vi "Threshold_Check.vi"(8 "error in (no error)":errorcluster, 11 "Simulators":T1 {"Milk Level" scale=0.0..100.0; "Bean Level" scale=0.0..100.0; "Water Level" scale=0.0..100.0}) -> (0 "error out":errorcluster, 2 "Success?":bool, 3 "Status":string)   [LabVIEW 2026]
uses:
  controls/Simulators.ctl
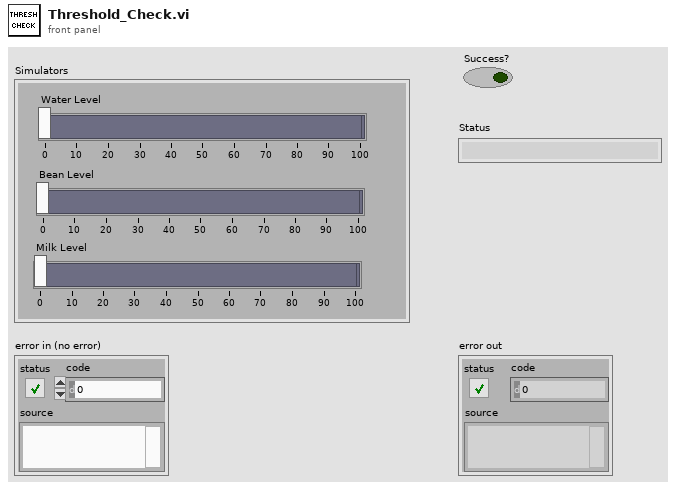
[diagram p1: front panel]
types:
  T1 = typedef "Simulators.ctl" = cluster{"Water Level":dbl, "Bean Level":dbl, "Milk Level":dbl}
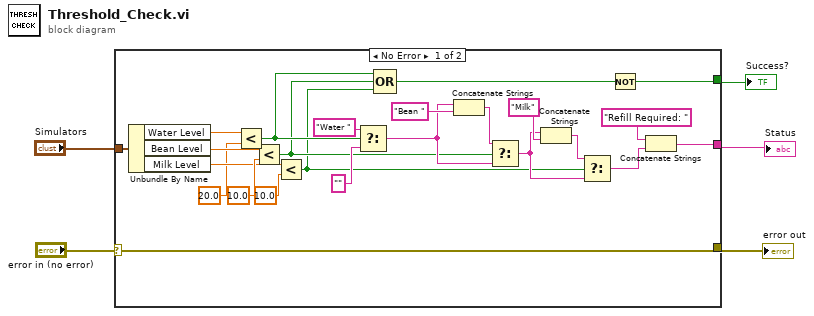
[diagram p0: block diagram]
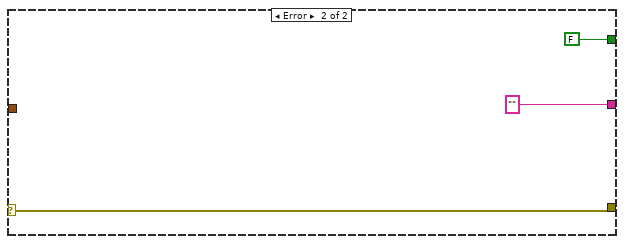
[diagram p2: hidden frame]
diagram:
  n1 = case shown="No Error" "error in (no error)" {
    selector: "error in (no error)" -> [w22 w32]
    tunnel: "Simulators" -> [w25 _]
    tunnel: [w22 w32] -> w3
    tunnel: [w11 ""] -> w2
    tunnel: [w6 FALSE] -> w1
    frame No Error {
      n2 = Unbundle By Name(w25) -> ("Water Level"=w24:dbl, "Bean Level"=w26:dbl, "Milk Level"=w27:dbl)
      n3 = Less?(x=w24, y=20.0) -> (x < y?=w10:bool)
      n4 = Less?(x=w26, y=10.0) -> (x < y?=w9:bool)
      n5 = Less?(x=w27, y=10.0) -> (x < y?=w8:bool)
      n6 = Select(t="Water " ("string"), s=w10, f="") -> (s? t:f=w16:string)
      n7 = Compound Arithmetic op=OR(w10, w9, w8) -> (w7:bool)
      n8 = Concatenate Strings(w16, "Bean " ("string")) -> (w17:string)
      n9 = Select(t=w17, s=w9, f=w16) -> (s? t:f=w13:string)
      n10 = Concatenate Strings(w13, "Milk" ("string")) -> (w14:string)
      n11 = Select(t=w14, s=w8, f=w13) -> (s? t:f=w12:string)
      n12 = Not(x=w7) -> (.not. x?=w6:bool)
      n13 = Concatenate Strings("Refill Required: " ("string"), w12) -> (w11:string)
    }
    frame Error {
    }
  }
  "Success?" <- w1
  "error out" <- w3
  "Status" <- w2
